vi "GetFactory&Floor.vi"(8 "error in (no error)":errorcluster caption="错误输入（无错误）", 10 "模式":enum16{"˜ÇŒÓ", "S^"}(ring), 11 "HttpClient 输入":refnum<class "HttpClient.lvclass"> caption="DNL_LabVIEW Object in") -> (0 "error out":errorcluster caption="错误输出", 1 "Data":string[][](array[string]), 3 "HttpClient 输出":refnum<class "HttpClient.lvclass"> caption="DNL_LabVIEW Object out")   [LabVIEW 2012, in "HttpClient.lvclass"]
uses:
  HttpClient.lvclass
  HttpClient.lvclass/HttpClient.ctl
  Libs/Http/Http.lvclass
  Libs/Http/Form.ctl
  Libs/Http/Method.ctl
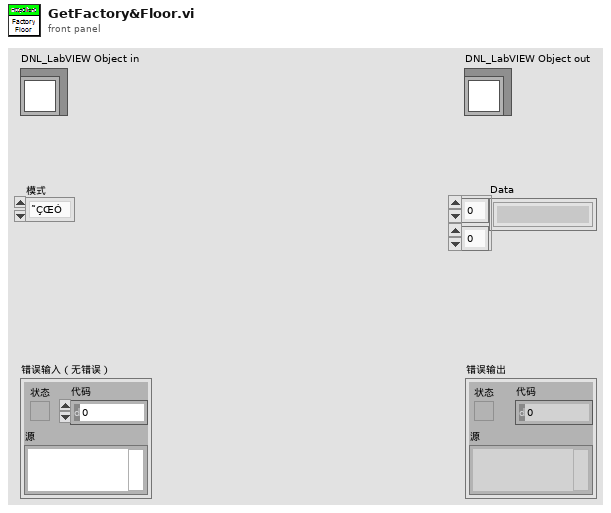
[diagram p1: front panel]
types:
  T1 = typedef "Http.lvclass/Form.ctl" = cluster{"±í†Î":string, "方法":T2}[]
  T2 = typedef "Http.lvclass/Method.ctl" = string
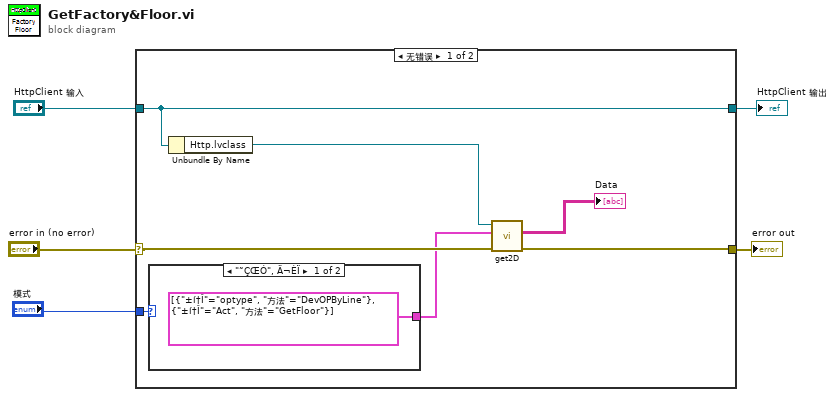
[diagram p0: block diagram]
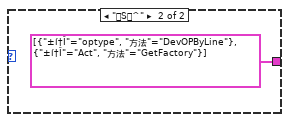
[diagram p2: hidden frame]
diagram:
  n1 = case shown="无错误" "error in (no error)" {
    selector: "error in (no error)" -> [w12 w16]
    tunnel: [w8 w16] -> w4
    tunnel: [w11 w15] -> w2
    tunnel: "HttpClient 输入" -> [w11 w15]
    tunnel: "模式" -> [w6 _]
    frame No Error {
      n2 = case shown="\"˜ÇŒÓ\", Ä¬ÈÏ" w6 {
        tunnel: [T1 [{"±í†Î"="optype", "方法"="DevOPByLine"}, {"±í†Î"="Act", "方法"="GetFloor"}] ("±í†Î") T1 [{"±í†Î"="optype", "方法"="DevOPByLine"}, {"±í†Î"="Act", "方法"="GetFactory"}] ("±í†Î")] -> w9
        frame "˜ÇŒÓ", Default {
        }
        frame "S^" {
        }
      }
      n3 = Unbundle By Name(w11) -> ("Http.lvclass"=w10:refnum<class "Http.lvclass">)
      n4 = call-dynamic "get2D.vi"("error in (no error)"=w12, "±í†Î"=w9, "HttpClient 输入"=w10) -> ("error out"=w8:errorcluster, "数组"=→"Data":string[][])  [unwired: 6 in, 1 out]
    }
    frame Error {
    }
  }
  "error out" <- w4
  "HttpClient 输出" <- w2
